vi "calSave.vi"(4 "O3 flow":dbl, 6 "save cal?":bool, 8 "m_660":dbl, 9 "m_532":dbl, 10 "Calibration":cluster{dbl[], dbl[]}[](graph), 11 "file path (dialog if empty)":path) -> ()   [LabVIEW 2011]
uses:
  <vilib>/Utility/file.llb/Write To Spreadsheet File (string).vi
  <vilib>/Utility/file.llb/Write To Spreadsheet File (DBL).vi
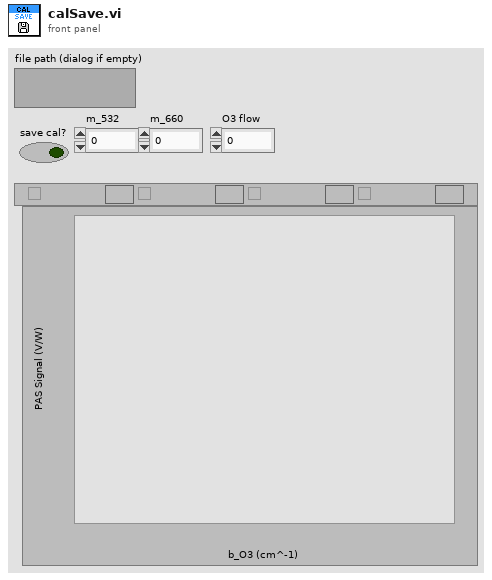
[diagram p1: front panel]
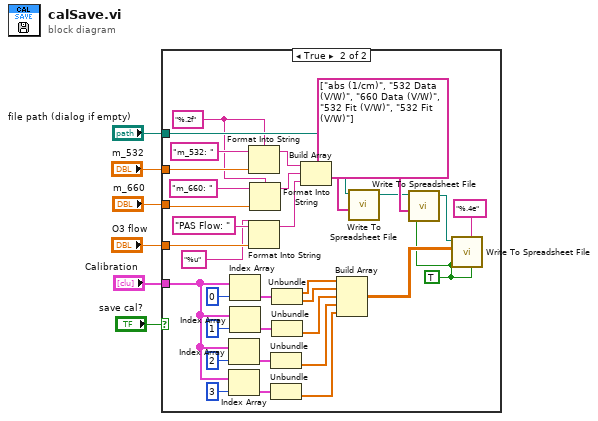
[diagram p0: block diagram]
diagram:
  n1 = case shown="True" "save cal?" {
    tunnel: "Calibration" -> [_ w35]
    tunnel: "file path (dialog if empty)" -> [_ w20]
    tunnel: "m_532" -> [_ w18]
    tunnel: "m_660" -> [_ w15]
    tunnel: "O3 flow" -> [_ w10]
    frame False {
    }
    frame True {
      w11 = "%.2f" ("format string")
      w21 = TRUE ("transpose? (no:F)")
      n2 = Index Array(array=w35, index=2) -> (element=w37:cluster{dbl[], dbl[]})
      n3 = Index Array(array=w35, index=3) -> (element=w36:cluster{dbl[], dbl[]})
      n4 = Index Array(array=w35, index=0) -> (element=w39:cluster{dbl[], dbl[]})
      n5 = Index Array(array=w35, index=1) -> (element=w38:cluster{dbl[], dbl[]})
      n6 = Format Into String(format string=w11, initial string="m_532: ", w18) -> (resulting string=w14:string)  [unwired: 1 in, 1 out]
      n7 = Format Into String(format string="%u", initial string="PAS Flow: ", w10) -> (resulting string=w8:string)  [unwired: 1 in, 1 out]
      n8 = Format Into String(format string=w11, initial string="m_660: ", w15) -> (resulting string=w13:string)  [unwired: 1 in, 1 out]
      n9 = Unbundle(w37) -> (w31:dbl[])  [unwired: 1 out]
      n10 = Unbundle(w36) -> (w30:dbl[])  [unwired: 1 out]
      n11 = Unbundle(w39) -> (w34:dbl[], w33:dbl[])
      n12 = Unbundle(w38) -> (w32:dbl[])  [unwired: 1 out]
      n13 = Build Array(w14, w13, w8) -> (w12:string[])
      n14 = Build Array(w34, w33, w32, w31, w30) -> (w29:dbl[][])
      n15 = call-poly <vilib>:"Write To Spreadsheet File.vi"("1D data"=w12, "file path (dialog if empty)"=w20) -> ("new file path (Not A Path if cancelled)"=w19:path)  [unwired: 6 in]
      n16 = call-poly <vilib>:"Write To Spreadsheet File.vi"("append to file? (new file:F)"=w21, "1D data"=string[] ["abs (1/cm)", "532 Data (V/W)", "660 Data (V/W)", "532 Fit (V/W)", "532 Fit (V/W)"], "file path (dialog if empty)"=w19) -> ("new file path (Not A Path if cancelled)"=w22:path)  [unwired: 5 in]
      n17 = call-poly <vilib>:"Write To Spreadsheet File.vi"("transpose? (no:F)"=w21, "format (%.3f)"="%.4e", "append to file? (new file:F)"=w21, "2D data"=w29, "file path (dialog if empty)"=w22) -> ()  [unwired: 3 in, 1 out]
    }
  }
